vi "Set Max Retries.vi"(8 "error in":errorcluster, 10 "Max Retries":u8=3, 11 "SDO Manager in":refnum<class "SDO Manager.lvclass">) -> (0 "error out":errorcluster, 3 "SDO Manager out":refnum<class "SDO Manager.lvclass">)   [LabVIEW 2020, in "SDO Manager.lvlib" / "SDO Manager.lvclass"]
uses:
  SDO Manager.lvclass
  SDO Manager.lvclass/SDO Manager.ctl
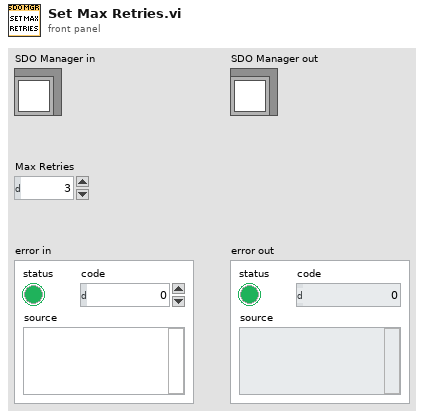
[diagram p1: front panel]
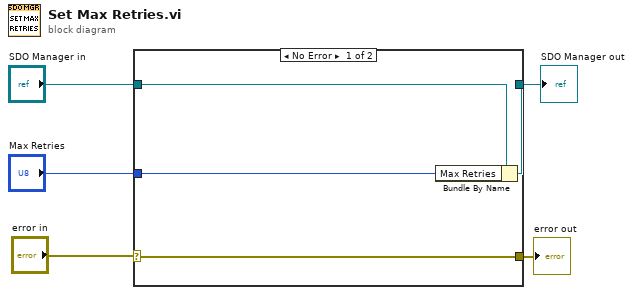
[diagram p0: block diagram]
diagram:
  n1 = case shown="No Error" "error in" {
    selector: "error in" -> [w9 w10]
    tunnel: [w9 w10] -> w2
    tunnel: [w7 w11] -> w4
    tunnel: "SDO Manager in" -> [w8 w11]
    tunnel: "Max Retries" -> [w6 _]
    frame No Error {
      n2 = Bundle By Name(cluster=w8, "Max Retries"=w6) -> (w7:refnum<class "SDO Manager.lvclass">)
    }
    frame Error {
    }
  }
  "error out" <- w2
  "SDO Manager out" <- w4
